vi "Get All Test Results.vi"(8 "error in (no error)":errorcluster, 11 "Test Result in":refnum<class "Test Result.lvclass">) -> (0 "error out":errorcluster, 2 "Test Results":T1[](array[typedef]), 3 "Test Result out":refnum<class "Test Result.lvclass">)   [LabVIEW 2013, in "Caraya.lvlib" / "Test Result.lvclass"]
uses:
  Test Result.lvclass
  Node Results.ctl
  Test Node.ctl
  Test Registration Data.ctl
  Assert Event Data.ctl
  Test Result.lvclass/Test Result.ctl
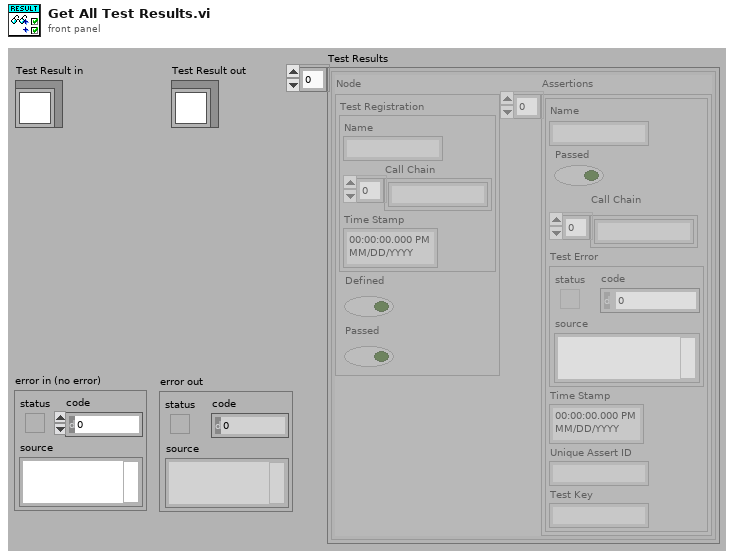
[diagram p1: front panel]
types:
  T1 = typedef "Caraya.lvlib/Test Result.lvclass/Node Results.ctl" = cluster{"Node":T2, "Assertions":T4[]}
  T2 = typedef "Caraya.lvlib/Test Result.lvclass/Test Node.ctl" = cluster{"Test Registration":T3, "Defined":bool, "Passed":bool}
  T3 = typedef "Caraya.lvlib/Test Result.lvclass/Test Registration Data.ctl" = cluster{"Name":string, "Call Chain":string[], "Time Stamp":timestamp}
  T4 = typedef "Caraya.lvlib/Test Result.lvclass/Assert Event Data.ctl" = cluster{"Name":string, "Passed":bool, "Call Chain":string[], "Test Error":errorcluster, "Time Stamp":timestamp, "Unique Assert ID":string, "Test Key":string}
  T5 = cluster{i32, string, "Time Stamp":timestamp, "Node Result":T1}
  T6 = cluster{i32, string, "Time Stamp":timestamp, "Node Result":T1}[]
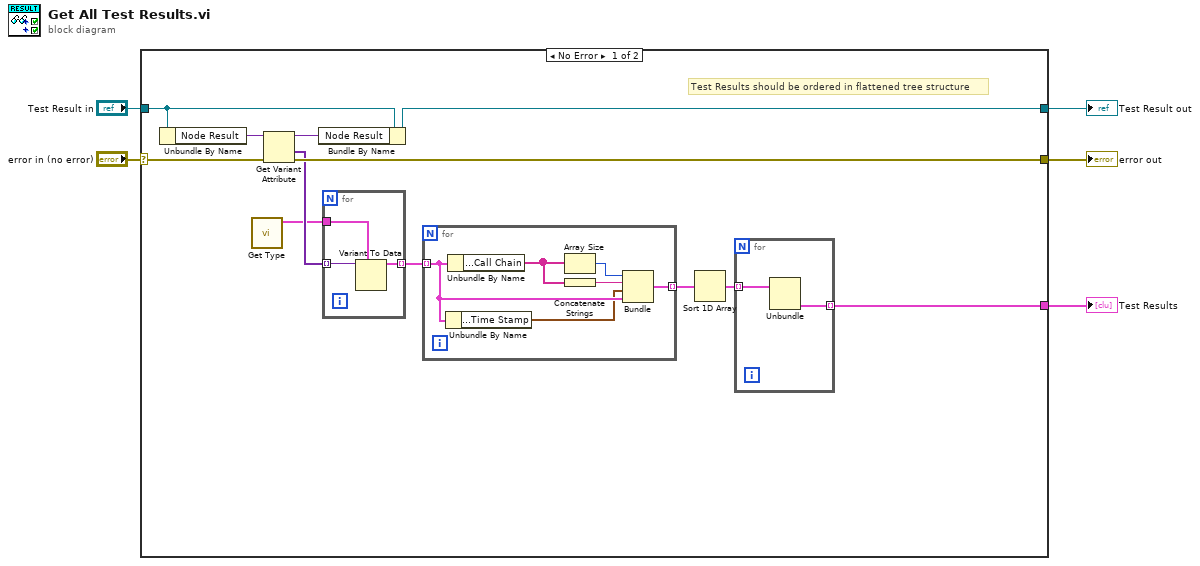
[diagram p0: block diagram]
diagram:
  n1 = case shown="No Error" "error in (no error)" {
    selector: "error in (no error)" -> [w12 w30]
    tunnel: [w13 w30] -> w4
    tunnel: [w16 w29] -> w2
    tunnel: "Test Result in" -> [w17 w29]
    tunnel: [w6 _] -> w1
    frame No Error {
      # "Test Results should be ordered in flattened tree structure"
      n2 = Unbundle By Name(w17) -> ("Node Result"=w15:variant)
      n3 = call "Get Type.vi"() -> ("Node Result"=w10:T1)  [unwired: 11 in]
      n4 = Get Variant Attribute(Variant=w15, error in=w12) -> (duplicate Variant=w14:variant, values=w11:variant[], error out=w13:errorcluster)  [unwired: 2 in, 1 out]
      n5 = Bundle By Name(cluster=w17, "Node Result"=w14) -> (w16:refnum<class "Test Result.lvclass">)
      n6 = for {
        tunnel: w11 -> [w28] mode=indexing
        tunnel: w10 -> [w27]
        tunnel: [w26] -> w8 mode=indexing
        n7 = Variant To Data(type=w27, Variant=w28) -> (data=w26:T1)  [unwired: 1 in, 1 out]
      }
      n8 = for {
        tunnel: w8 -> [w22] mode=indexing
        tunnel: [w25] -> w9 mode=indexing
        n9 = Unbundle By Name(w22) -> ("Node.Test Registration.Time Stamp"=w21:timestamp)
        n10 = Unbundle By Name(w22) -> ("Node.Test Registration.Call Chain"=w24:string[])
        n11 = Array Size(array=w24) -> (size(s)=w20:i32)
        n12 = Concatenate Strings(w24) -> (w23:string)
        n13 = Bundle(w20, w23, "Time Stamp"=w21, "Node Result"=w22) -> (w25:T5)  [unwired: 1 in]
      }
      n14 = Sort 1D Array(array=w9) -> (sorted array=w7:T6)
      n15 = for {
        tunnel: w7 -> [w19] mode=indexing
        tunnel: [w18] -> w6 mode=indexing
        n16 = Unbundle(w19) -> ("Node Result"=w18:T1)  [unwired: 3 out]
      }
    }
    frame Error {
    }
  }
  "error out" <- w4
  "Test Result out" <- w2
  "Test Results" <- w1
